vi "Py Convert.vi"(8 "error in (no error)":errorcluster, 11 "configuration scripts":path) -> (0 "error out":errorcluster, 3 "I2C Commands":u16[][](array[numeric]))   [LabVIEW 2025, in "I2C Bus Monitor.lvclass"]
uses:
  I2C Bus Monitor.lvclass
  <vilib>/Utility/error.llb/Trim Whitespace One-Sided.vi
  I2C Bus Monitor.lvclass/I2C Bus Monitor.ctl
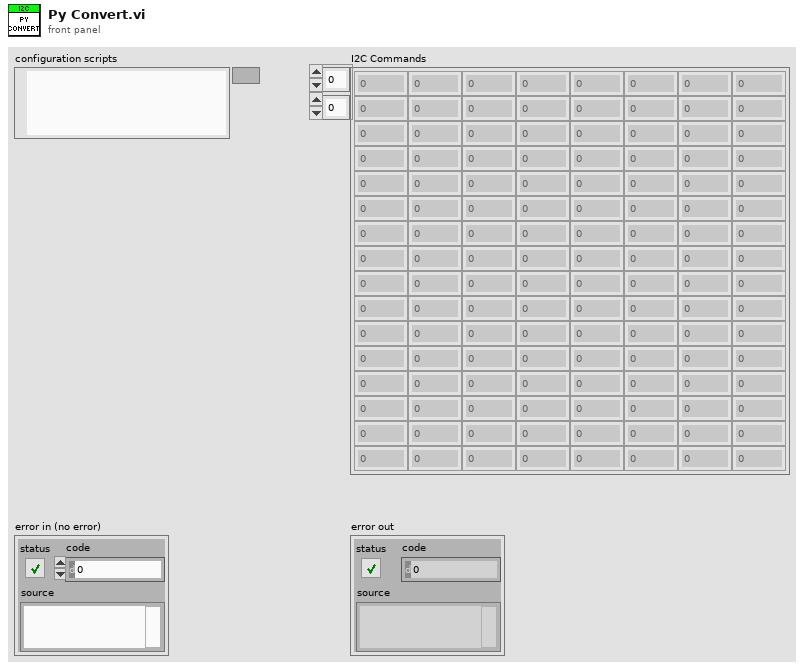
[diagram p1: front panel]
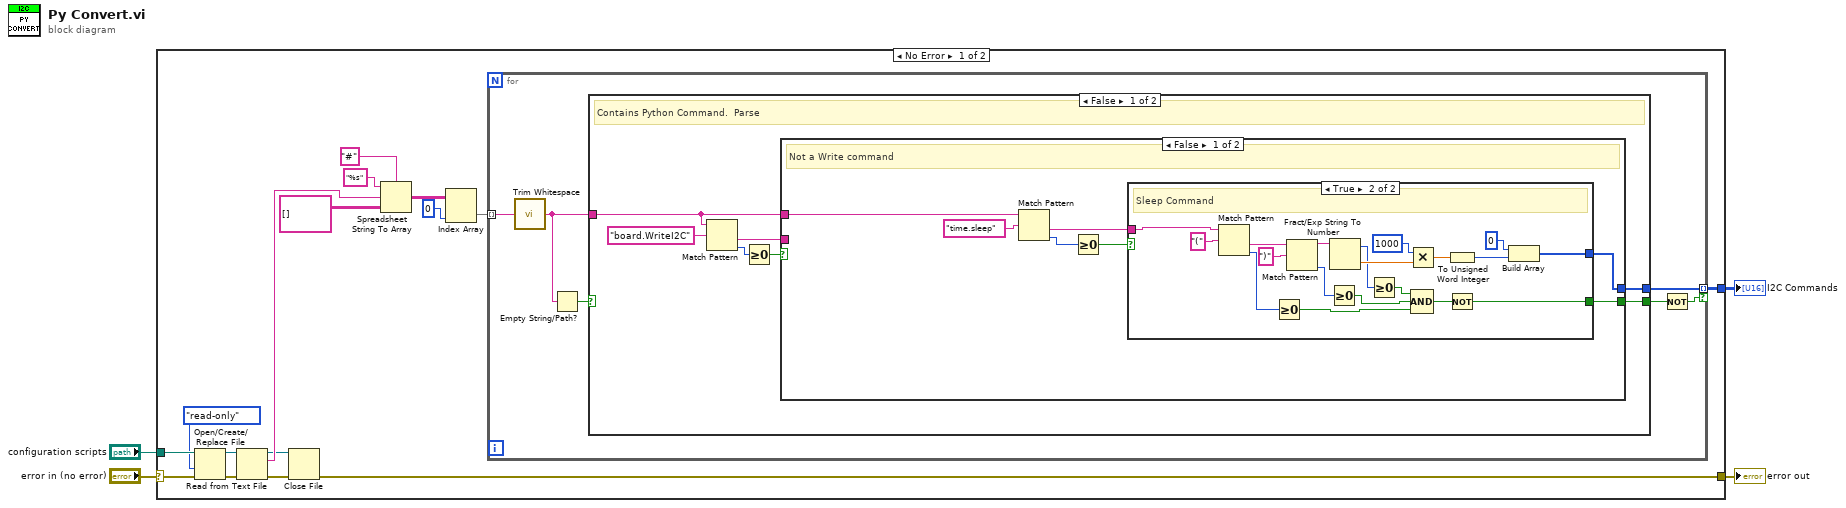
[diagram p0: block diagram]
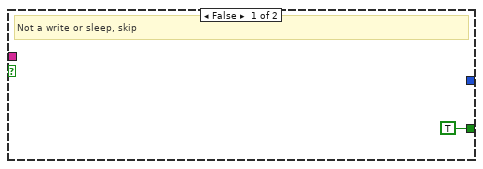
[diagram p2: hidden frame]
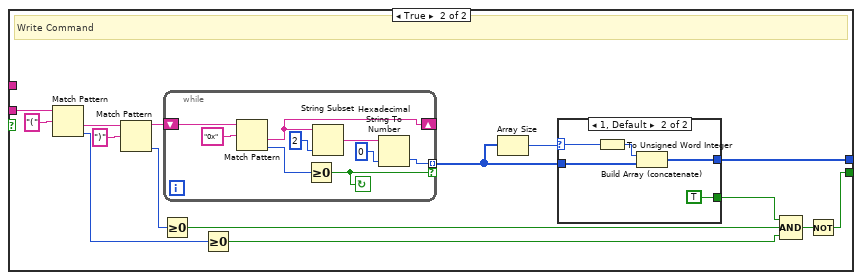
[diagram p3: hidden frame]
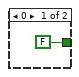
[diagram p4: hidden frame]
diagram:
  n1 = case shown="No Error" "error in (no error)" {
    selector: "error in (no error)" -> [w18 w92]
    tunnel: [w20 w92] -> w4
    tunnel: "configuration scripts" -> [w19 _]
    tunnel: [w17 _] -> w1
    frame No Error {
      n2 = Open/Create/Replace File(file path (use dialog)=w19, error in=w18, access (0:read/write)=enum16{"read/write", "read-only", "write-only"}."read-only") -> (refnum out=w9:refnum<file>, error out=w10:errorcluster)  [unwired: 3 in, 1 out]
      n3 = Read from Text File(file (use dialog)=w9, error in=w10) -> (refnum out=w11:refnum<file>, text=w13:string, error out=w12:errorcluster)  [unwired: 2 in, 1 out]
      n4 = Close File(refnum=w11, error in=w12) -> (error out=w20:errorcluster)  [unwired: 1 out]
      n5 = Spreadsheet String To Array(delimiter (Tab)="#", format string="%s", spreadsheet string=w13, array type (2D Dbl)=string[][] []) -> (array=w8:string[][])
      n6 = Index Array(array=w8, index (col)=0 ("disabled index (col)")) -> (element=w6:string[])  [unwired: 1 in]
      n7 = for {
        tunnel: [w21] -> w17 mode=indexing if=w23
        tunnel: w6 -> [w22] mode=indexing
        n8 = call <vilib>:"Trim Whitespace.vi"("string"=w22) -> ("trimmed string"=w25:string)  [unwired: 1 in]
        n9 = Empty String/Path?(string/path=w25) -> (empty?=w26:bool)
        n10 = case shown="False" w26 {
          selector: w26 -> [_ w91]
          tunnel: [w28 w91] -> w24
          tunnel: w25 -> [w29 _]
          tunnel: [w27 _] -> w21
          frame False {
            # "Contains Python Command.  Parse"
            n11 = Match Pattern(string=w29, regular expression="board.WriteI2C") -> (after substring=w30:string, offset past match=w31:i32)  [unwired: 1 in, 2 out]
            n12 = Greater Or Equal To 0?(x=w31) -> (x >= 0?=w32:bool)
            n13 = case shown="False" w32 {
              tunnel: w30 -> [_ w67]
              tunnel: [w34 w62] -> w27
              tunnel: w29 -> [w39 _]
              tunnel: [w36 w66] -> w28
              frame False {
                # "Not a Write command"
                n14 = Match Pattern(string=w39, regular expression="time.sleep") -> (after substring=w35:string, offset past match=w38:i32)  [unwired: 1 in, 2 out]
                n15 = Greater Or Equal To 0?(x=w38) -> (x >= 0?=w37:bool)
                n16 = case shown="True" w37 {
                  tunnel: [TRUE w49] -> w36
                  tunnel: w35 -> [_ w60]
                  tunnel: [_ w43] -> w34
                  frame False {
                    # "Not a write or sleep, skip"
                  }
                  frame True {
                    # "Sleep Command"
                    n17 = Match Pattern(string=w60, regular expression="(") -> (after substring=w59:string, offset past match=w56:i32)  [unwired: 1 in, 2 out]
                    n18 = Greater Or Equal To 0?(x=w56) -> (x >= 0?=w51:bool)
                    n19 = Match Pattern(string=w59, regular expression=")") -> (before substring=w54:string, offset past match=w55:i32)  [unwired: 1 in, 2 out]
                    n20 = Greater Or Equal To 0?(x=w55) -> (x >= 0?=w52:bool)
                    n21 = Fract/Exp String To Number(string=w54) -> (offset past number=w42:i32, number=w47:dbl)  [unwired: 3 in]
                    n22 = Greater Or Equal To 0?(x=w42) -> (x >= 0?=w53:bool)
                    n23 = Multiply(x=1000, y=w47) -> (x*y=w46:dbl)
                    n24 = Compound Arithmetic op=AND(w53, w52, w51) -> (w50:bool)
                    n25 = To Unsigned Word Integer(number=w46) -> (unsigned 16bit integer=w45:u16)
                    n26 = Not(x=w50) -> (.not. x?=w49:bool)
                    n27 = Build Array(u16 0 ("element"), w45) -> (w43:u16[])
                  }
                }
              }
              frame True {
                # "Write Command"
                n28 = Match Pattern(string=w67, regular expression="(") -> (after substring=w75:string, offset past match=w72:i32)  [unwired: 1 in, 2 out]
                n29 = Match Pattern(string=w75, regular expression=")") -> (before substring=w65:string, offset past match=w71:i32)  [unwired: 1 in, 2 out]
                n30 = Greater Or Equal To 0?(x=w71) -> (x >= 0?=w70:bool)
                n31 = while {
                  shift-right: [w84] -> _
                  shift-left: w65 -> [w89]
                  tunnel: [w83] -> w63 mode=indexing if=w82
                  stop <- w82 continue-if-true
                  n32 = Match Pattern(string=w89, regular expression="0x") -> (after substring=w84:string, offset past match=w88:i32)  [unwired: 1 in, 2 out]
                  n33 = Greater Or Equal To 0?(x=w88) -> (x >= 0?=w82:bool)
                  n34 = String Subset(string=w84, length (rest)=2 ("length (rest)")) -> (substring=w85:string)  [unwired: 1 in]
                  n35 = Hexadecimal String To Number(string=w85, default (0uL)=u16 0 ("default (0 I32)")) -> (number=w83:u16)  [unwired: 1 in, 1 out]
                }
                n36 = Greater Or Equal To 0?(x=w72) -> (x >= 0?=w69:bool)
                n37 = Array Size(array=w63) -> (size(s)=w64:i32)
                n38 = case shown="1, Default" w64 {
                  selector: w64 -> [_ w80]
                  tunnel: w63 -> [_ w81]
                  tunnel: [_ w78] -> w62
                  tunnel: [FALSE TRUE] -> w61
                  frame 0 {
                  }
                  frame 1, Default {
                    n39 = To Unsigned Word Integer(number=w80) -> (unsigned 16bit integer=w79:u16)
                    n40 = Build Array (concatenate)(w79, w81) -> (w78:u16[])
                  }
                }
                n41 = Compound Arithmetic op=AND(w61, w70, w69) -> (w68:bool)
                n42 = Not(x=w68) -> (.not. x?=w66:bool)
              }
            }
          }
          frame True {
            # "Comment Line, do nothing"
          }
        }
        n43 = Not(x=w24) -> (.not. x?=w23:bool)
      }
    }
    frame Error {
    }
  }
  "error out" <- w4
  "I2C Commands" <- w1
